vi "Caracterizacion_bn.vi"() -> ()   [LabVIEW 2017]
uses:
  EnumEstados1.ctl
  <vilib>/Analysis/3filter.llb/Filter Passband Type.ctl
  <vilib>/Analysis/baseanly.llb/IIR Cascade Filter (DBL).vi
  <vilib>/Analysis/NI_AALBase.lvlib
  <vilib>/Utility/NIReport.llb/NI_report.lvclass
  <vilib>/addons/_office/NI_ReportGenerationToolkit.lvlib
  <vilib>/addons/_office/excel.llb/Excel Easy Table (str).vi
panel:
  out "Array out":cluster{"Array":dbl[], "Array out":dbl[]}[](graph)
  out "Voltaje de corte":dbl
  out "Resistencia":dbl[](array[numeric])
  out "Potencia":dbl[](array[numeric])
  in  "Numeric Control":dbl=0.01 format="%.2f"
  in  "order":i32=2
  in  "Stop Button":bool
  in  "Blank Button 2":bool
  in  "Blank Button":bool
  out "Eficiencia:":dbl
  out "Factor de Llenado:":dbl
  in  "Ok":bool
  in  "Save Button":bool
  in  "Guardar en:":path
  in  "Dispositivo:":enum16{"OLED", "OFET", "OPV"}(ring)
  in  "Voltaje final:":dbl
  in  "Voltaje inicial:":dbl
  out "Voltage-Current Characterization:":cluster{dbl[], "Filtered X":dbl[]}(graph)
  in  "Paso":dbl
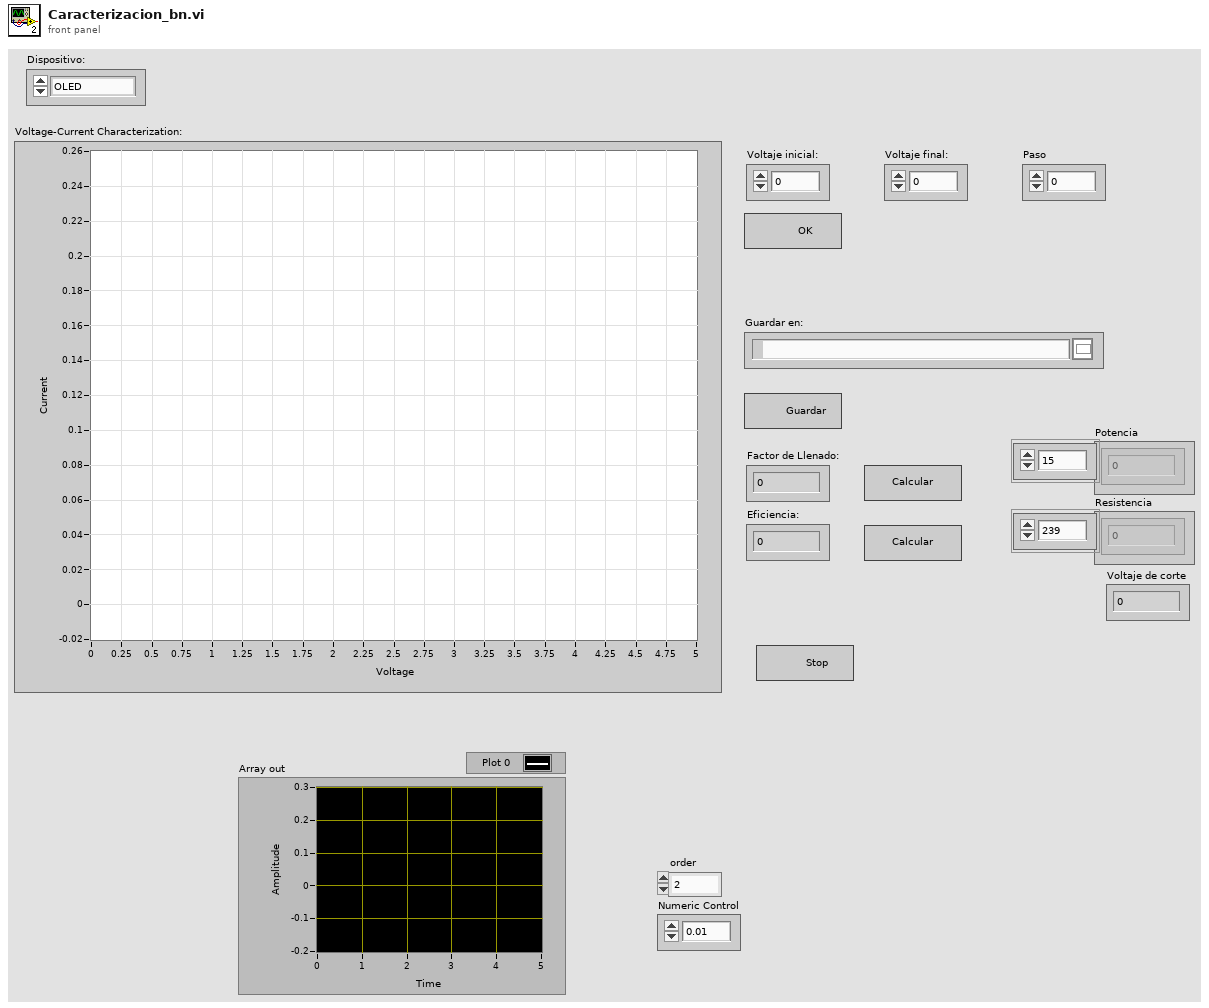
[diagram p1: front panel]
types:
  T1 = typedef "EnumEstados1.ctl" = enum16{"Inicio", "LecturaDatos", "Cierre"}
  T2 = typedef "NI_AALBase.lvlib/Filter Passband Type.ctl" = enum32{"Lowpass", "Highpass", "Bandpass", "Bandstop"}
  T3 = enum16{"Standard Report", "HTML", "Word", "Excel"}
  T4 = enum16{"maximized", "minimized", "normal", "no change"}
  T5 = enum16{"open", "open or create", "create or replace", "create", "open (read-only)"}
  T6 = cluster{"task out":refnum<k21>, "error out":errorcluster}
  T7 = cluster{"filter structure":enum32{"IIR 2nd Order", "IIR 4th Order"}, "Reverse Coefficients":dbl[], "Forward Coefficients":dbl[]}
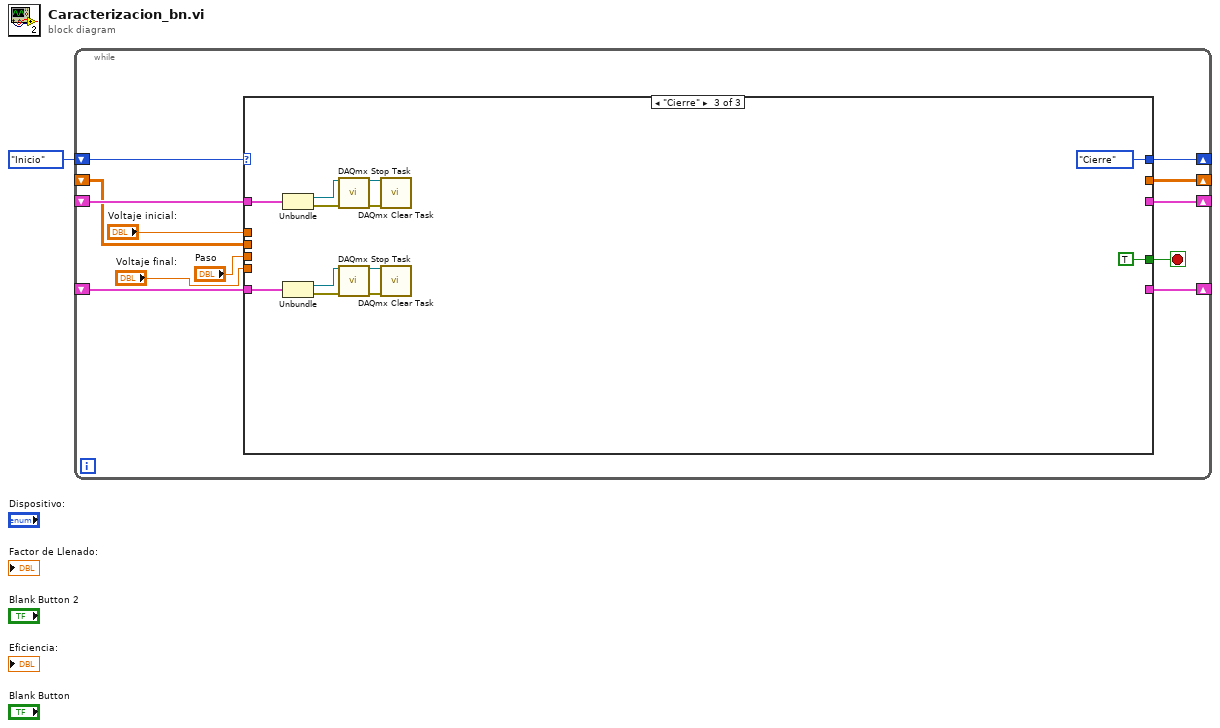
[diagram p0: block diagram]
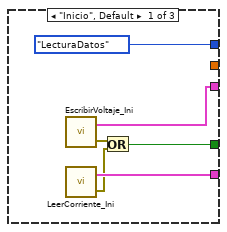
[diagram p2: hidden frame]
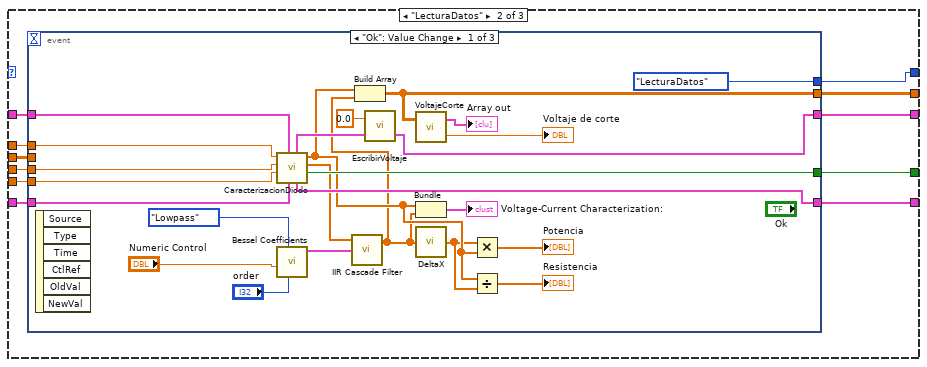
[diagram p3: hidden frame]
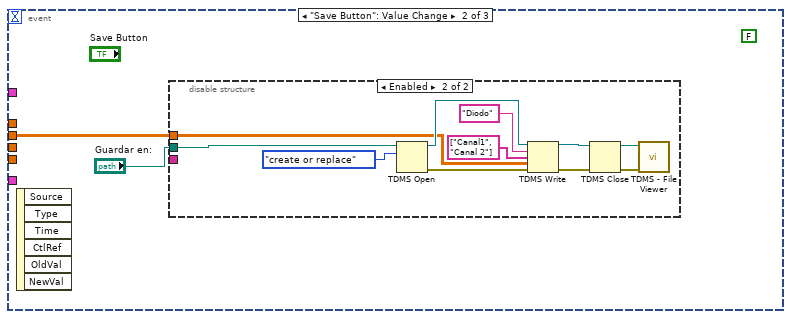
[diagram p4: hidden frame]
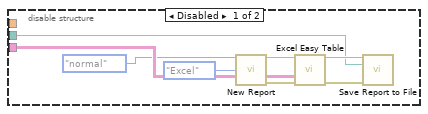
[diagram p5: hidden frame]
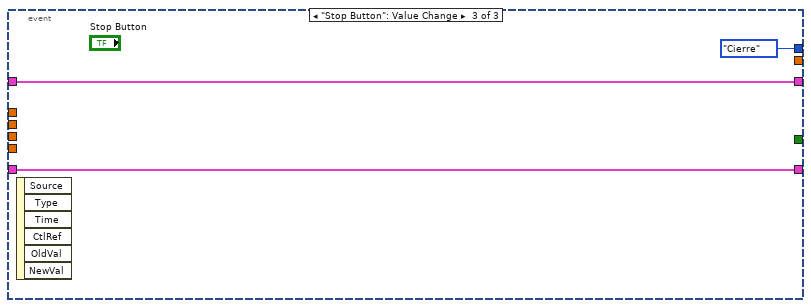
[diagram p6: hidden frame]
diagram:
  n1 = while {
    shift-right: [w5] -> _
    shift-left: EnumEstados1."Inicio" -> [w13]
    shift-right: [w9] -> _
    shift-left: _ -> [w8]
    shift-right: [w7] -> _
    shift-left: _ -> [w6]
    shift-right: [w4] -> _
    shift-left: _ -> [w3]
    stop <- w2 stop-if-true
    n2 = case shown="\"Cierre\"" w13 {
      tunnel: "Voltaje final:" -> [_ w30 _]
      tunnel: "Voltaje inicial:" -> [_ w24 _]
      tunnel: "Paso" -> [_ w25 _]
      tunnel: [w18 w28 _] -> w9
      tunnel: w8 -> [_ w29 w87]
      tunnel: [w17 w26 _] -> w7
      tunnel: w6 -> [_ w27 w86]
      tunnel: [EnumEstados1."LecturaDatos" w23 EnumEstados1."Cierre"] -> w5
      tunnel: [_ w22 _] -> w4
      tunnel: w3 -> [_ w21 _]
      tunnel: [w14 w20 TRUE] -> w2
      frame "Inicio", Default {
        n3 = call "EscribirVoltaje_Ini.vi"() -> ("error out"=w16:errorcluster, "cluster"=w18:T6)  [unwired: 2 in]
        n4 = call "LeerCorriente_Ini.vi"() -> ("error out"=w15:errorcluster, "output cluster"=w17:T6)  [unwired: 2 in]
        n5 = Or(x=w16, y=w15) -> (x .or. y?=w14:bool)
      }
      frame "LecturaDatos" {
        n6 = event shown="[0] \"Ok\": Value Change" {
          selector: _ -> [_ _ _]
          dyn-events: _ -> [_ _ _]
          timeout: _ -> [_ _ _]
          tunnel: w30 -> [w46 _ _]
          tunnel: w29 -> [w45 _ w79]
          tunnel: [w51 _ w79] -> w28
          tunnel: w27 -> [w44 _ w78]
          tunnel: [w42 _ w78] -> w26
          tunnel: w25 -> [w47 _ _]
          tunnel: w24 -> [w48 _ _]
          tunnel: [EnumEstados1."LecturaDatos" _ EnumEstados1."Cierre"] -> w23
          tunnel: [w39 _ _] -> w22
          tunnel: w21 -> [_ w56 _]
          tunnel: [w40 _ _] -> w20
          event "Ok": Value Change {
            n7 = event-data() -> ()  [unwired: 1 in, 6 out]
            n8 = call "CaracterizacionDiodo.vi"("Corriente"=w44, "Voltaje"=w45, "Voltaje final:"=w46, "Paso"=w47, "Voltaje inicial:"=w48) -> ("Error?"=w40:bool, 2:"Corriente"=w38:dbl[], 3:"Voltaje"=w36:dbl[], 4:"Corriente"=w42:T6, 5:"Voltaje"=w43:T6)  [unwired: 2 in]
            n9 = call <vilib>:"Bessel Coefficients.vi"("order"="order", "filter type"=Filter_Passband_Type."Lowpass", "low cutoff freq: fl"="Numeric Control") -> ("IIR Filter Cluster"=w54:T7)  [unwired: 7 in, 1 out]
            n10 = call-poly <vilib>:"IIR Cascade Filter.vi"("IIR Filter Cluster"=w54, "X"=w38) -> ("Filtered X"=w31:dbl[])  [unwired: 1 in, 1 out]
            n11 = Build Array(w36, w31) -> (w39:dbl[][])
            n12 = call "EscribirVoltaje.vi"("cluster"=w43, "data"=0.0) -> ("Cluster"=w51:T6)  [unwired: 1 out]
            n13 = call "VoltajeCorte.vi"("Array in"=w39) -> ("Voltaje de corte"=→"Voltaje de corte":dbl, "Array out"=→"Array out":cluster{"Array":dbl[], "Array out":dbl[]}[])  [unwired: 1 in]
            n14 = Bundle("Voltaje"=w36, "Filtered X"=w31) -> (→"Voltage-Current Characterization:":cluster{"Voltaje":dbl[], "Filtered X":dbl[]})  [unwired: 1 in]
            n15 = call "DeltaX.vi"("Array in"=w31) -> ("Array out"=w35:dbl[])
            n16 = Multiply(x=w35, y=w36) -> (x*y=→"Potencia":dbl[])
            n17 = Divide(x=w36, y=w35) -> (x/y=→"Resistencia":dbl[])
          }
          event "Save Button": Value Change {
            (unwired) FALSE
            n18 = event-data() -> ()  [unwired: 1 in, 6 out]
            n19 = disable-structure shown="Enabled" {
              disable-tunnel: _ -> [w63 _]
              disable-tunnel: "Guardar en:" -> [w58 w69]
              disable-tunnel: w56 -> [_ w66]
              frame Disabled {
                n20 = call <vilib>:"New Report.vi"("window state (normal)"=T4."normal", "report type"=T3."Excel") -> ("report out"=w65:refnum<class "NI_report.lvclass">, "error out"=w64:errorcluster)  [unwired: 12 in]
                n21 = call-poly <vilib>:"Excel Easy Table.vi"("report in"=w65, "text data"=w63, "error in (no error)"=w64) -> ("report out"=w62:refnum<class "NI_report.lvclass">, "error out"=w61:errorcluster)  [unwired: 8 in, 3 out]
                n22 = call-dynamic "Save Report to File.vi"("report in"=w62, "report file path"=w58, "error in (no error)"=w61) -> ()  [unwired: 11 in, 2 out]
              }
              frame Enabled {
                n23 = TDMS Open(10:T5."create or replace" ("operation (0:open)"), 11:w69) -> (0:w73:errorcluster, 3:w70:refnum<k34>)  [unwired: 5 in]
                n24 = TDMS Write(0:w70, 5:"Diodo" ("group name in (Untitled)"), 7:string[] ["Canal1", "Canal 2"] ("channel name(s) in (Untitled)"), 9:w66, 11:w73) -> (4:w71:refnum<k34>, 15:w72:errorcluster)  [unwired: 1 in, 2 out]
                n25 = TDMS Close(8:w72, 11:w71) -> (0:w68:errorcluster, 3:w67:path)
                n26 = call <vilib>:"TDMS - File Viewer.vi"("error in (no error)"=w68, "file path"=w67) -> ()  [unwired: 4 in, 2 out]
              }
            }
          }
          event "Stop Button": Value Change {
            n27 = event-data() -> ()  [unwired: 1 in, 6 out]
          }
        }
      }
      frame "Cierre" {
        n28 = Unbundle(w87) -> ("task out"=w85:refnum<k21>, "error out"=w84:errorcluster)
        n29 = Unbundle(w86) -> ("task out"=w83:refnum<k21>, "error out"=w82:errorcluster)
        n30 = call <vilib>:"DAQmx Stop Task.vi"("task/channels in"=w85, "error in"=w84) -> ("task out"=w91:refnum<k21>, "error out"=w90:errorcluster)  [unwired: 12 in]
        n31 = call <vilib>:"DAQmx Stop Task.vi"("task/channels in"=w83, "error in"=w82) -> ("task out"=w89:refnum<k21>, "error out"=w88:errorcluster)  [unwired: 12 in]
        n32 = call <vilib>:"DAQmx Clear Task.vi"("task in"=w91, "error in"=w90) -> ()  [unwired: 13 in, 1 out]
        n33 = call <vilib>:"DAQmx Clear Task.vi"("task in"=w89, "error in"=w88) -> ()  [unwired: 13 in, 1 out]
      }
    }
  }
